vi "GC EX Helium - Step 1.vi"(7 "Step":i32, 8 "error in":errorcluster, 9 "Test Results In":T8, 10 "Gas":T1, 11 "GC Configuration":T2) -> (0 "error out":errorcluster, 1 "Test Results Out":T8, 2 "Gas Out":T1 caption="Gas", 3 "GC Configuration Out":T2)   [LabVIEW 2015]
uses:
  Controls/Test Information.ctl
  Controls/Vacuum Test.ctl
  Controls/Test Timing.ctl
  Controls/Vaccum Thresholds.ctl
  Controls/Helium Test.ctl
  Controls/Helium Thresholds.ctl
  CAN Communication/Gas/Typedefs/Session Handle.ctl
  CAN Communication/Gas/Gas.lvclass
  Controls/Test Results.ctl
  Controls/Step Result.ctl
  SubVIs/Timing/Timing.lvlib
panel:
  out "NI-DAQ Pressure":dbl
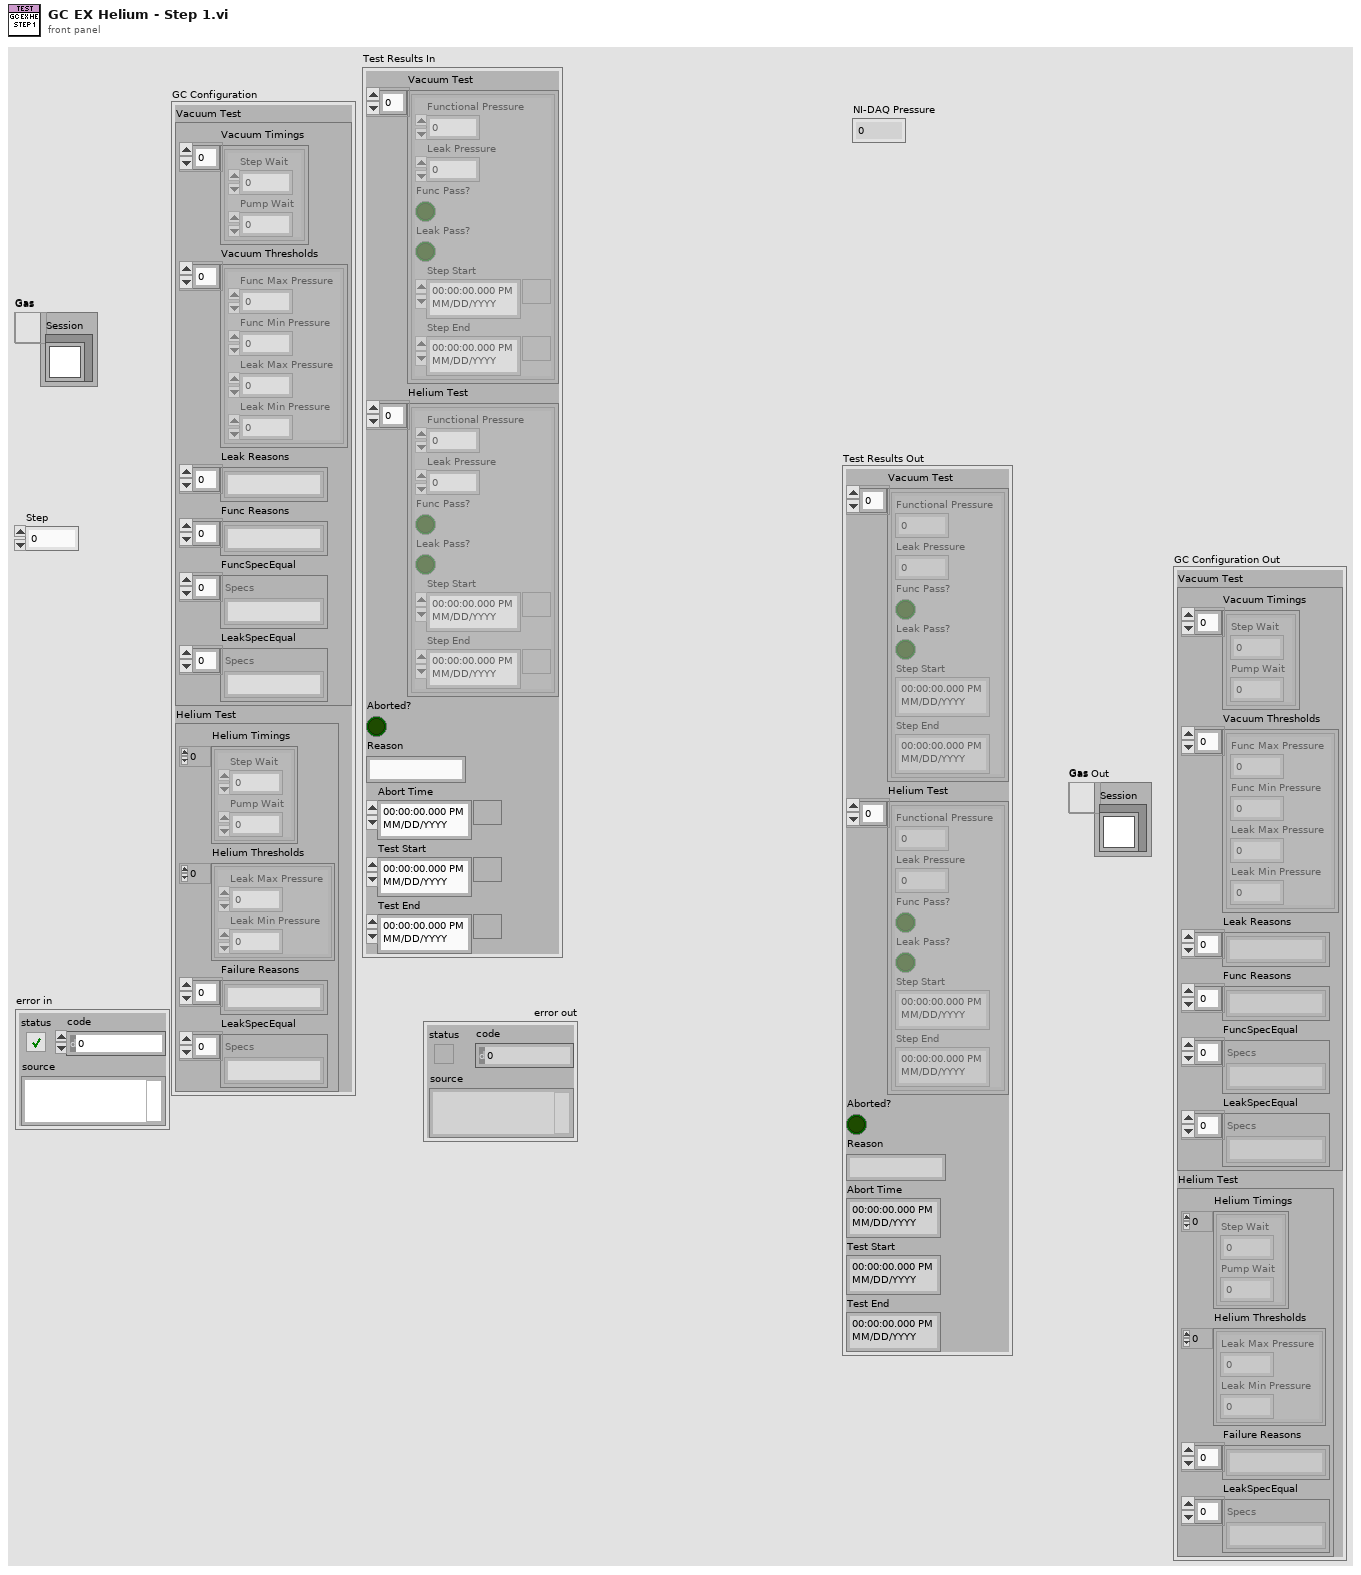
[diagram p1: front panel]
types:
  T1 = typedef "Gas.lvclass/Session Handle.ctl" = refnum<data-value>
  T2 = typedef "Test Information.ctl" = cluster{"Vacuum Test":T3, "Helium Test":T6}
  T3 = typedef "Vacuum Test.ctl" = cluster{"Vacuum Timings":T4[], "Vacuum Thresholds":T5[], "Leak Reasons":string[], "Func Reasons":string[], "FuncSpecEqual":string[], "LeakSpecEqual":string[]}
  T4 = typedef "Test Timing.ctl" = cluster{"Step Wait":dbl, "Pump Wait":dbl}
  T5 = typedef "Vaccum Thresholds.ctl" = cluster{"Func Max Pressure":dbl, "Func Min Pressure":dbl, "Leak Max Pressure":dbl, "Leak Min Pressure":dbl}
  T6 = typedef "Helium Test.ctl" = cluster{"Helium Timings":T4[], "Helium Thresholds":T7[], "Failure Reasons":string[], "LeakSpecEqual":string[]}
  T7 = typedef "Helium Thresholds.ctl" = cluster{"Leak Max Pressure":dbl, "Leak Min Pressure":dbl}
  T8 = typedef "Test Results.ctl" = cluster{"Vacuum Test":T9[], "Helium Test":T9[], "Aborted?":bool, "Reason":string, "Abort Time":timestamp, "Test Start":timestamp, "Test End":timestamp}
  T9 = typedef "Step Result.ctl" = cluster{"Functional Pressure":dbl, "Leak Pressure":dbl, "Func Pass?":bool, "Leak Pass?":bool, "Step Start":timestamp, "Step End":timestamp}
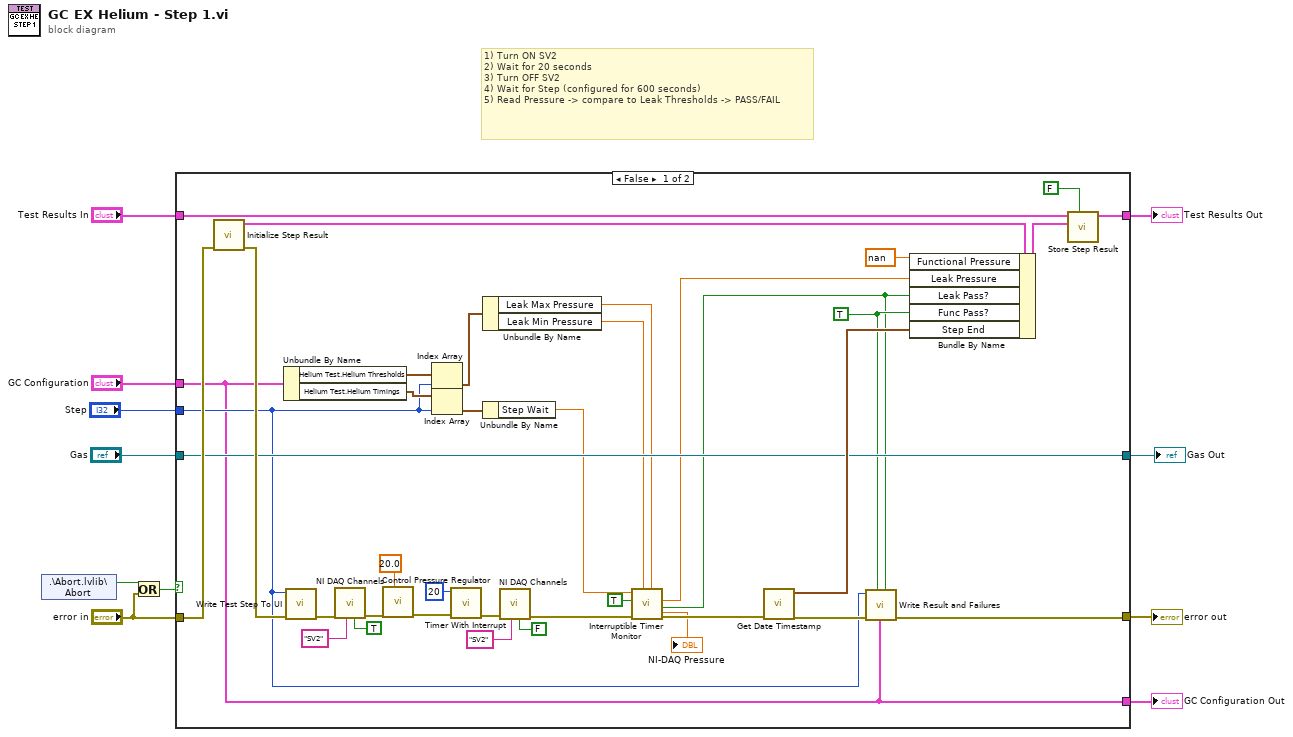
[diagram p0: block diagram]
diagram:
  # "1) Turn ON SV2\n2) Wait for 20 seconds\n3) Turn OFF SV2\n4) Wait for Step (configured for 600 seconds)\n5) Read Pressure -> compare to Leak Thresholds -> PASS/FAIL"
  n1 = shared-variable ".\\Abort.lvlib\\Abort"() -> (w10:bool)  [unwired: 1 in, 1 out]
  n2 = Or(x=w10, y="error in") -> (x .or. y?=w9:bool)
  n3 = case shown="False" w9 {
    tunnel: "error in" -> [w49 w52]
    tunnel: "Test Results In" -> [w46 w53]
    tunnel: [w47 w53] -> w7
    tunnel: [w36 w52] -> w6
    tunnel: "GC Configuration" -> [w34 w51]
    tunnel: "Step" -> [w35 _]
    tunnel: [w34 w51] -> w3
    tunnel: [w39 w50] -> w1
    tunnel: "Gas" -> [w39 w50]
    frame False {
      w31 = TRUE ("Func Pass?")
      n4 = call "Initialize Step Result.vi"("error in (no error)"=w49) -> ("error out"=w48:errorcluster, "New Step Result"=w45:T9)  [unwired: 8 in, 1 out]
      n5 = Unbundle By Name(w34) -> ("Helium Test.Helium Thresholds"=w42:T7[], "Helium Test.Helium Timings"=w41:T4[])
      n6 = call "Write Test Step To UI.vi"("error in (no error)"=w48, "Step"=w35) -> ("error out"=w24:errorcluster)  [unwired: 9 in]
      n7 = call "NI DAQ Channels.vi"("Control"=TRUE ("State"), "Channel"="SV2", "error in (no error)"=w24) -> ("error out"=w27:errorcluster)  [unwired: 7 in, 1 out]
      n8 = call "Control Pressure Regulator.vi"("error in"=w27, "Desired PSI"=20.0) -> ("error out"=w25:errorcluster)  [unwired: 8 in, 1 out]
      n9 = Index Array(array=w42, index=w35) -> (element=w38:T7)
      n10 = Index Array(array=w41, index=w35) -> (element=w40:T4)
      n11 = call "Timer With Interrupt.vi"("error in (no error)"=w25, "Wait (s)"=20) -> ("error out"=w23:errorcluster)  [unwired: 7 in, 2 out]
      n12 = Unbundle By Name(w38) -> ("Leak Max Pressure"=w18:dbl, "Leak Min Pressure"=w19:dbl)
      n13 = Unbundle By Name(w40) -> ("Step Wait"=w21:dbl)
      n14 = call "NI DAQ Channels.vi"("Control"=FALSE ("State"), "Channel"="SV2", "error in (no error)"=w23) -> ("error out"=w22:errorcluster)  [unwired: 7 in, 1 out]
      n15 = call "Interruptible Timer Monitor.vi"("Max"=w18, "Min"=w19, "error in (no error)"=w22, "Update UI?"=TRUE, "Wait (s)"=w21) -> ("error out"=w16:errorcluster, "In Range?"=w15:bool, "Leak Rate"=w17:dbl, "NI-DAQ Pressure"=→"NI-DAQ Pressure":dbl)  [unwired: 2 in, 1 out]
      n16 = call "Get Date Timestamp.vi"("error in (no error)"=w16) -> ("error out"=w37:errorcluster, "current time"=w43:timestamp)  [unwired: 9 in]
      n17 = call "Write Result and Failures.vi"("Leak"=w15, "GC Configuration"=w34, "Func"=w31, "error in (no error)"=w37, "Step"=w35) -> ("error out"=w36:errorcluster)  [unwired: 6 in]
      n18 = Bundle By Name(cluster=w45, "Functional Pressure"=nan, "Leak Pressure"=w17, "Leak Pass?"=w15, "Func Pass?"=w31, "Step End"=w43) -> (w44:T9)
      n19 = call "Store Step Result.vi"("Vacuum?"=FALSE, "Step Result"=w44, "Test Results In"=w46) -> ("Test Results Out"=w47:T8)  [unwired: 8 in]
    }
    frame True {
    }
  }
  "error out" <- w6
  "Test Results Out" <- w7
  "GC Configuration Out" <- w3
  "Gas Out" <- w1
